vi "ActionVIOnDownload - Set Scan Rate.vi"(5 "System Definition Dir":path, 6 "IP address":string, 7 "Details Ref":refnum<vi>, 8 "error in (no error)":errorcluster, 10 "WebDAV session in":T1, 11 "Device Item Ref in":T2 format="%.0x") -> (0 "error out":errorcluster, 2 "WebDAV session out":T1, 3 "Device Item Ref out":T2 format="%.0x")   [LabVIEW 2016, in "Scan Engine Custom Device.lvlib"]
uses:
  Scan Engine Custom Device.lvlib
  <vilib>/NI Veristand/Custom Device API/Custom Device API.lvlib
  Globals/Property Strings.vi
  <vilib>/NI Veristand/Custom Device API/Custom Device Item Ref.ctl
  <vilib>/WebDAVClient/Advanced/SessionHandle.ctl
  <vilib>/WebDAVClient/NI_WebDAV.lvlib
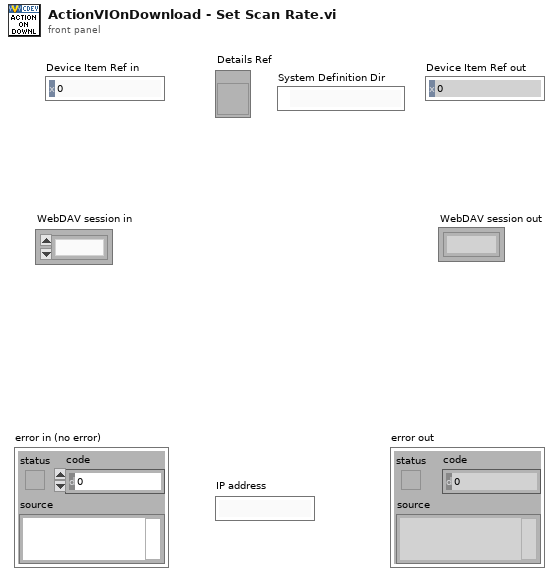
[diagram p1: front panel]
types:
  T1 = typedef "NI_WebDAV.lvlib/SessionHandle.ctl" = refnum<k1>
  T2 = typedef "Custom Device API.lvlib/Custom Device Item Ref.ctl" = u64
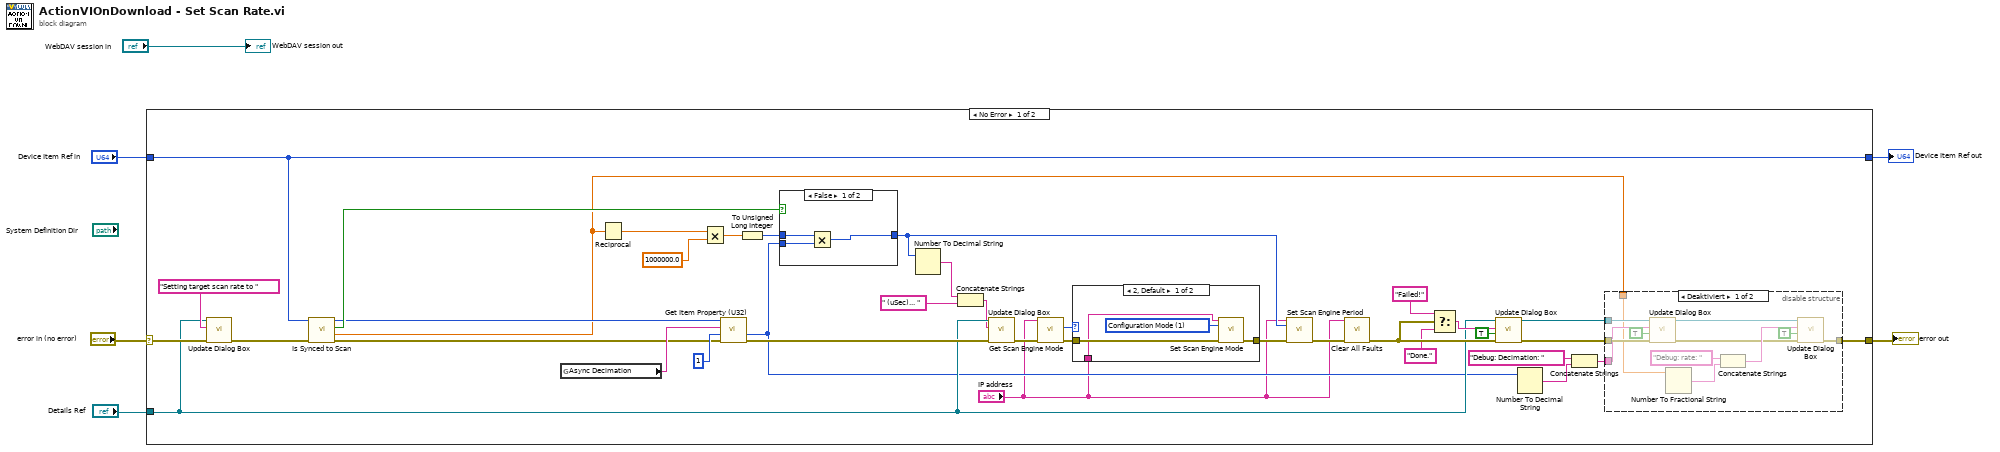
[diagram p0: block diagram]
diagram:
  n1 = case shown="No Error" "error in (no error)" {
    selector: "error in (no error)" -> [w35 w68]
    tunnel: [w13 w68] -> w1
    tunnel: "Device Item Ref in" -> [w32 w67]
    tunnel: [w32 w67] -> w2
    tunnel: "Details Ref" -> [w25 _]
    frame No Error {
      n2 = call "Update Dialog Box.vi"("error in (no error)"=w35, "Text to add"="Setting target scan rate to ", "Details Ref in"=w25) -> ("error out"=w33:errorcluster)  [unwired: 7 in, 1 out]
      n3 = call "Is Synced to Scan.vi"("error in"=w33, "Item Ref in"=w32) -> ("error out"=w10:errorcluster, "Engine Rate"=w8:dbl, "Sync to Scan?"=w36:bool, "Item Ref out"=w9:T2)  [unwired: 6 in]
      n4 = global read "Property Strings.vi" "Async Decimation"() -> (w40:string)
      n5 = Reciprocal(x=w8) -> (1/x=w12:dbl)
      n6 = Multiply(x=w12, y=1000000.0) -> (x*y=w39:dbl)
      n7 = call <vilib>:"Get Item Property (U32).vi"("error in (no error)"=w10, "Default Value"=u32 1, "Property Name"=w40, "Item Ref in"=w9) -> ("error out"=w26:errorcluster, "Value"=w17:u32)  [unwired: 4 in, 2 out]
      n8 = To Unsigned Long Integer(number=w39) -> (unsigned 32bit integer=w11:u32)
      n9 = case shown="False" w36 {
        tunnel: w11 -> [w65 w66]
        tunnel: w17 -> [w64 _]
        tunnel: [w63 w66] -> w23
        frame False {
          n10 = Multiply(x=w65, y=w64) -> (x*y=w63:u32)
        }
        frame True {
        }
      }
      n11 = Number To Decimal String(number=w23) -> (decimal integer string=w21:string)  [unwired: 1 in]
      n12 = Concatenate Strings(w21, " (uSec)... ") -> (w24:string)
      n13 = call "Update Dialog Box.vi"("error in (no error)"=w26, "Text to add"=w24, "Details Ref in"=w25) -> ("error out"=w22:errorcluster)  [unwired: 7 in, 1 out]
      n14 = call <vilib>:"Get Scan Engine Mode.vi"("error in (no error)"=w22, "target address (localhost)"="IP address") -> ("error out"=w42:errorcluster, "mode"=w43:i32)  [unwired: 8 in]
      n15 = case shown="2, Default" w43 {
        tunnel: w42 -> [w60 w62]
        tunnel: [w59 w62] -> w44
        tunnel: "IP address" -> [w58 _]
        frame 2, Default {
          w61 = 1 items=["Configuration Mode"=1, "Active Mode"=2] ("mode (Active Mode)")
          n16 = call <vilib>:"Set Scan Engine Mode.vi"("target address (localhost)"=w58, "mode (Active Mode)"=w61, "error in (no error)"=w60) -> ("error out"=w59:errorcluster)  [unwired: 12 in]
        }
        frame 1 {
        }
      }
      n17 = call <vilib>:"Set Scan Engine Period.vi"("target address (localhost)"="IP address", "scan period (uSec)"=w23, "error in (no error)"=w44) -> ("error out"=w37:errorcluster)  [unwired: 12 in]
      n18 = call <vilib>:"Clear All Faults.vi"("error in (no error)"=w37, "target address (localhost)"="IP address") -> ("error out"=w31:errorcluster)  [unwired: 9 in]
      n19 = Select(t="Failed!" ("Text to add"), s=w31, f="Done." ("Text to add")) -> (s? t:f=w29:string)
      n20 = call "Update Dialog Box.vi"("error in (no error)"=w31, "Add EOL? (F)"=TRUE, "Text to add"=w29, "Details Ref in"=w25) -> ("error out"=w19:errorcluster, "Details Ref out"=w18:refnum<vi>)  [unwired: 6 in]
      n21 = Number To Decimal String(number=w17) -> (decimal integer string=w15:string)  [unwired: 1 in]
      n22 = Concatenate Strings("Debug: Decimation: " ("string"), w15) -> (w14:string)
      n23 = disable-structure shown="Deaktiviert" {
        disable-tunnel: w19 -> [w55 w57]
        disable-tunnel: w18 -> [w54 _]
        disable-tunnel: w14 -> [w53 _]
        disable-tunnel: [w46 w57] -> w13
        disable-tunnel: w8 -> [w45 _]
        frame Disabled {
          n24 = call "Update Dialog Box.vi"("error in (no error)"=w55, "Add EOL? (F)"=TRUE, "Text to add"=w53, "Details Ref in"=w54) -> ("error out"=w48:errorcluster, "Details Ref out"=w47:refnum<vi>)  [unwired: 6 in]
          n25 = Number To Fractional String(number=w45) -> (F-format string=w51:string)  [unwired: 3 in]
          n26 = Concatenate Strings("Debug: rate: " ("string"), w51) -> (w52:string)
          n27 = call "Update Dialog Box.vi"("error in (no error)"=w48, "Add EOL? (F)"=TRUE, "Text to add"=w52, "Details Ref in"=w47) -> ("error out"=w46:errorcluster)  [unwired: 6 in, 1 out]
        }
        frame Enabled {
        }
      }
    }
    frame Error {
    }
  }
  "error out" <- w1
  "Device Item Ref out" <- w2
  "WebDAV session out" <- "WebDAV session in"
